vi "Copy UI Files Into Destination.vi"(8 "error in":errorcluster, 10 "user interface details":T1[](array[typedef]), 11 "destination path":path) -> (0 "error out":errorcluster)   [LabVIEW 2020, in "Measurement Plugin Measurement Server.lvlib"]
uses:
  Measurement Plugin Measurement Server.lvlib
  TypeDefs/User Interface Details.ctl
  Build Assets/User Interface Type.ctl
  <vilib>/ErrorRing/Error Ring.xnode
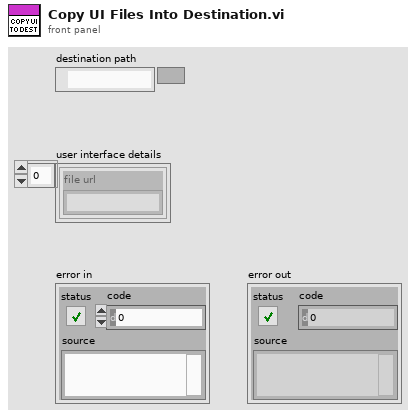
[diagram p1: front panel]
types:
  T1 = typedef "Measurement Plugin Measurement Server.lvlib/User Interface Details.ctl" = cluster{"file url":string}
  T2 = typedef "Measurement Plugin Measurement Server.lvlib/User Interface Type.ctl" = enum16{"Loose VI", "VI in lvlib", "VI in lvlibp"}
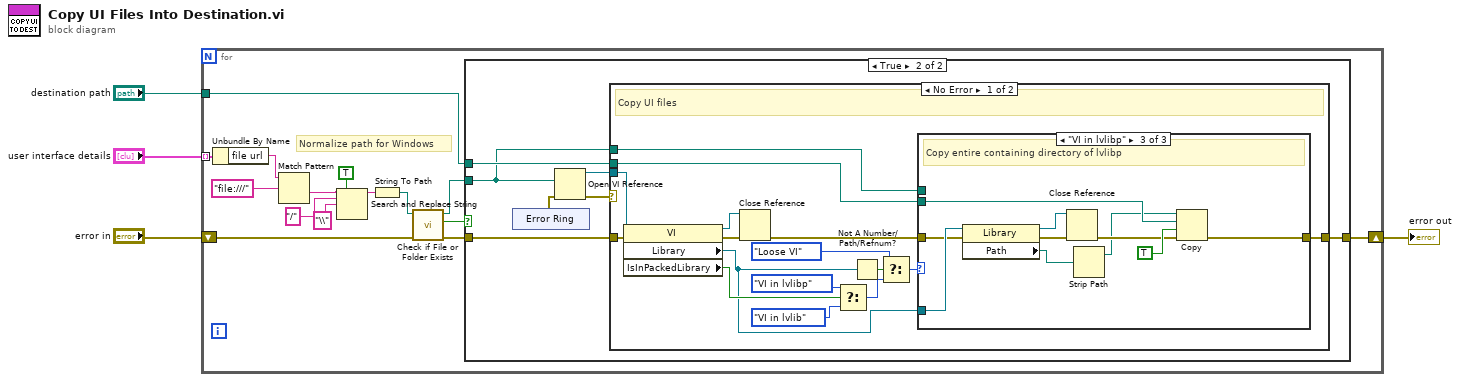
[diagram p0: block diagram]
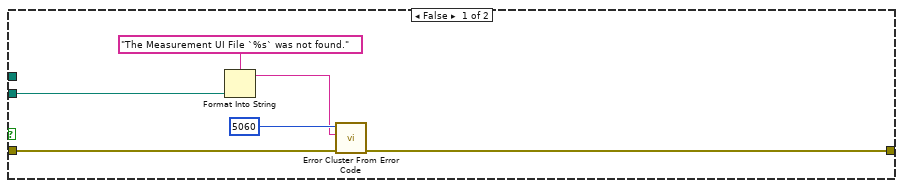
[diagram p2: hidden frame]
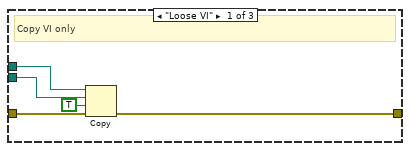
[diagram p3: hidden frame]
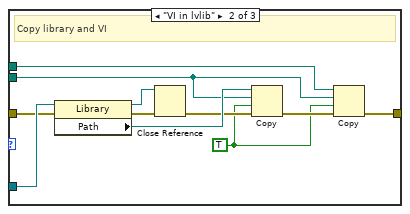
[diagram p4: hidden frame]
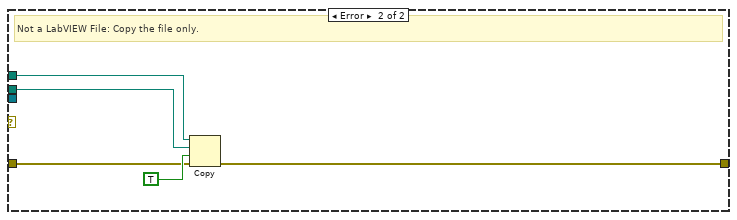
[diagram p5: hidden frame]
diagram:
  n1 = for {
    tunnel: "destination path" -> [w15]
    tunnel: "user interface details" -> [w18] mode=indexing
    shift-right: [w19] -> w2
    shift-left: "error in" -> [w14]
    # "Normalize path for Windows"
    n2 = Unbundle By Name(w18) -> ("file url"=w16:string)
    n3 = Match Pattern(string=w16, regular expression="file:///") -> (after substring=w9:string)  [unwired: 1 in, 3 out]
    n4 = Search and Replace String(replace all?=TRUE ("replace all? (F)"), input string=w9, search string="/" ("after substring"), replace string="\\" ("after substring")) -> (result string=w8:string)  [unwired: 4 in, 3 out]
    n5 = String To Path(string=w8) -> (path=w12:path)
    n6 = call <vilib>:"Check if File or Folder Exists.vi"("error in (no error)"=w14, "path"=w12) -> ("error out"=w13:errorcluster, "file or folder exists?"=w10:bool, "dup path"=w11:path)  [unwired: 7 in]
    n7 = case shown="True" w10 {
      tunnel: [w23 w32] -> w19
      tunnel: w15 -> [_ w28]
      tunnel: w13 -> [w24 w27]
      tunnel: w11 -> [w21 w26]
      frame False {
        n8 = Format Into String(format string="The Measurement UI File `%s` was not found." ("error message (\"\")"), w21) -> (resulting string=w20:string)  [unwired: 2 in, 1 out]
        n9 = call <vilib>:"Error Cluster From Error Code.vi"("error in (no error)"=w24, "error message (\"\")"=w20, "error code (0)"=5060) -> ("error out"=w23:errorcluster)  [unwired: 6 in]
      }
      frame True {
        n10 = xnode "Error Ring"() -> ("error out"=w31:errorcluster)
        n11 = Open VI Reference(vi path=w26, error in (no error)=w31) -> (vi reference=w29:refnum<vi>, error out=w30:errorcluster)  [unwired: 4 in]
        n12 = case shown="No Error" w30 {
          tunnel: w27 -> [w48 w79]
          tunnel: [w46 w78] -> w32
          tunnel: w29 -> [w49 _]
          tunnel: w28 -> [w45 w77]
          tunnel: w26 -> [w44 w76]
          frame No Error {
            # "Copy UI files"
            n13 = property class="VI"(reference=w49, error in=w48) -> (reference out=w42:refnum<vi>, error out=w47:errorcluster, "Library"=w34:refnum<vi>, "IsInPackedLibrary"=w39:bool)
            n14 = Close Reference(reference=w42, error in (no error)=w47) -> (error out=w43:errorcluster)
            n15 = Select(t=User_Interface_Type."VI in lvlibp", s=w39, f=User_Interface_Type."VI in lvlib") -> (s? t:f=w36:T2)
            n16 = Not A Number/Path/Refnum?(number/path/refnum=w34) -> (NaN/Path/Refnum?=w41:bool)
            n17 = Select(t=User_Interface_Type."Loose VI", s=w41, f=w36) -> (s? t:f=w35:T2)
            n18 = case shown="\"VI in lvlibp\"" w35 {
              tunnel: [w50 w58 w68] -> w46
              tunnel: w34 -> [_ w65 w75]
              tunnel: w43 -> [w54 w64 w74]
              tunnel: w45 -> [w53 w56 w69]
              tunnel: w44 -> [w52 w57 _]
              frame "Loose VI" {
                # "Copy VI only"
                n19 = Copy(8:w54, 9:TRUE ("overwrite (F)"), 10:w53, 11:w52) -> (0:w50:errorcluster)  [unwired: 1 in, 2 out]
              }
              frame "VI in lvlib" {
                w55 = TRUE ("overwrite (F)")
                # "Copy library and VI"
                n20 = property class="Library"(reference=w65, error in=w64) -> (reference out=w60:refnum<vi>, error out=w62:errorcluster, "Path"=w63:path)
                n21 = Close Reference(reference=w60, error in (no error)=w62) -> (error out=w61:errorcluster)
                n22 = Copy(8:w61, 9:w55, 10:w56, 11:w63) -> (0:w59:errorcluster)  [unwired: 1 in, 2 out]
                n23 = Copy(8:w59, 9:w55, 10:w56, 11:w57) -> (0:w58:errorcluster)  [unwired: 1 in, 2 out]
              }
              frame "VI in lvlibp" {
                # "Copy entire containing directory of lvlibp"
                n24 = property class="Library"(reference=w75, error in=w74) -> (reference out=w70:refnum<vi>, error out=w72:errorcluster, "Path"=w67:path)
                n25 = Close Reference(reference=w70, error in (no error)=w72) -> (error out=w71:errorcluster)
                n26 = Strip Path(path=w67) -> (stripped path=w66:path)  [unwired: 1 out]
                n27 = Copy(8:w71, 9:TRUE ("overwrite (F)"), 10:w69, 11:w66) -> (0:w68:errorcluster)  [unwired: 1 in, 2 out]
              }
            }
          }
          frame Error {
            # "Not a LabVIEW File: Copy the file only."
            n28 = Copy(8:w79, 9:TRUE ("overwrite (F)"), 10:w77, 11:w76) -> (0:w78:errorcluster)  [unwired: 1 in, 2 out]
          }
        }
      }
    }
  }
  "error out" <- w2
